vi "DB_LeeEstadoEquipos.vi"(8 "error in (no error)":errorcluster, 11 "db in":T1) -> (0 "error out":errorcluster, 2 "ESTADO_EQUIPOS":string[](array[string]), 3 "db out":T1)   [LabVIEW 2018]
uses:
  <vilib>/addons/database/Connection.llb/Conn ObjectReference.ctl
  <vilib>/Utility/sysdir.llb/System Directory Type.ctl
  <vilib>/Utility/file.llb/Read Delimited Spreadsheet (string).vi
  <vilib>/addons/database/Connection.llb/Conn Execute.vi
  <vilib>/addons/database/Recordset.llb/Rec Fetch Recordset Data (R).vi
  <vilib>/addons/database/Recordset.llb/Rec Destroy - Connection.vi
  <vilib>/addons/database/_DB Variant To Data/Database Variant To Data.xnode
  <vilib>/addons/database/NI_Database_API.lvlib
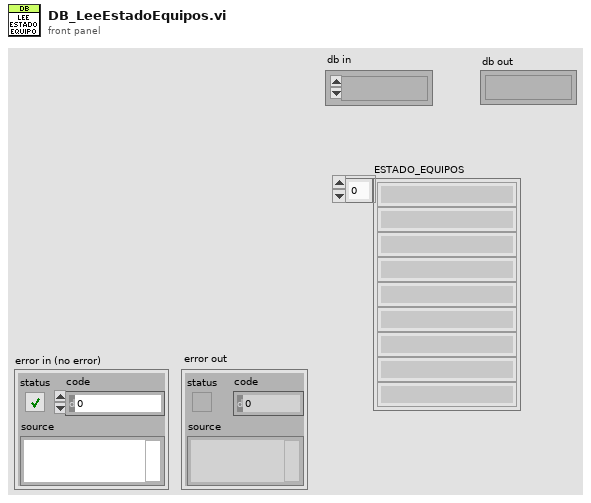
[diagram p1: front panel]
types:
  T1 = typedef "NI_Database_API.lvlib/Conn ObjectReference.ctl" = refnum<k1>
  T2 = typedef "System Directory Type.ctl" = i32
  T3 = typedef "NI_Database_API.lvlib/Rec ObjectReference.ctl" = refnum<k1>
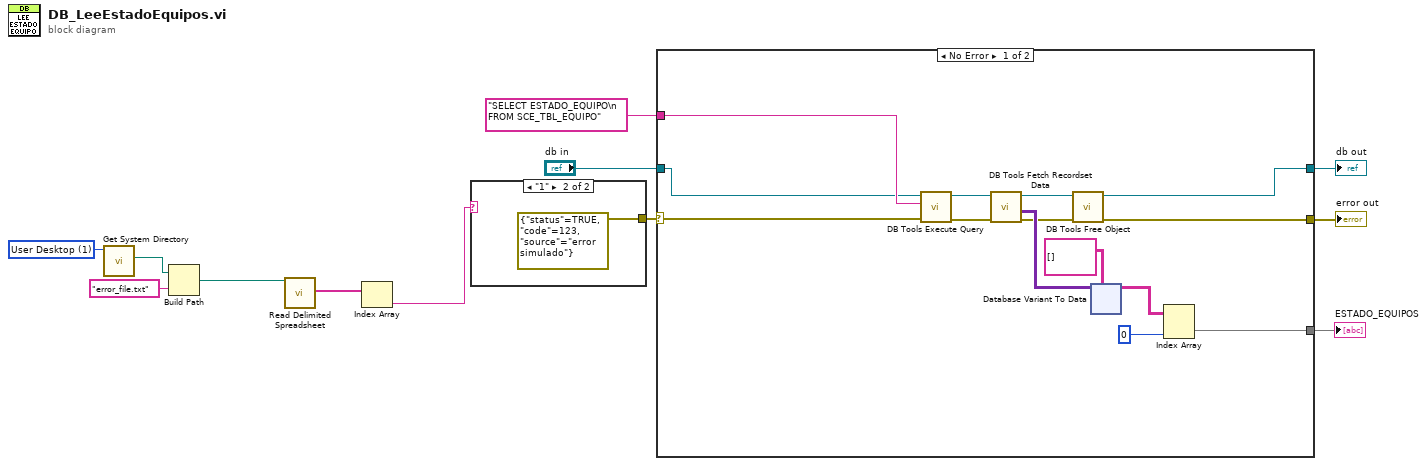
[diagram p0: block diagram]
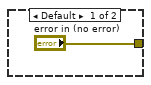
[diagram p2: hidden frame]
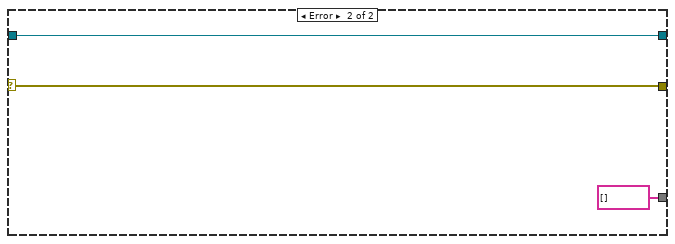
[diagram p3: hidden frame]
diagram:
  w7 = T2 1 items=["User Home"=0, "User Desktop"=1, "User Documents"=2, "User Application Data"=3, "User Preferences"=4, "User Temporary"=5, "Public Documents"=6, "Public Application Data"=7, "Public Preferences"=8, "Public Cache"=13, "System Core Libraries"=9, "System Installed Libraries"=10, "Application Files"=11, "Boot Volume Root"=12] ("system directory type")
  n1 = call <vilib>:"Get System Directory.vi"("system directory type"=w7) -> ("system directory"=w6:path)  [unwired: 10 in]
  n2 = Build Path(base path=w6, name or relative path="error_file.txt") -> (appended path=w4:path)
  n3 = call-poly <vilib>:"Read Delimited Spreadsheet.vi"("file path (dialog if empty)"=w4) -> ("first row"=w3:string[])  [unwired: 9 in, 5 out]
  n4 = Index Array(array=w3) -> (element=w2:string)  [unwired: 1 in]
  n5 = case shown="\"1\"" w2 {
    tunnel: ["error in (no error)" errorcluster {"status"=TRUE, "code"=123, "source"="error simulado"} ("error in (error)")] -> w11
    frame Default {
    }
    frame "1" {
    }
  }
  n6 = case shown="No Error" w11 {
    selector: w11 -> [w26 w75]
    tunnel: [w28 w75] -> w12
    tunnel: "SELECT ESTADO_EQUIPO\n  FROM SCE_TBL_EQUIPO" ("SQL") -> [w25 _]
    tunnel: "db in" -> [w15 w74]
    tunnel: [w17 w74] -> w8
    tunnel: [w16 string[] [] ("data")] -> w1
    frame No Error {
      n7 = call-poly <vilib>:"DB Tools Execute Query.vi"("error in (no error)"=w26, "SQL query"=w25, "connection reference"=w15) -> ("error out"=w27:errorcluster, "recordset reference"=w24:T3)  [unwired: 5 in]
      n8 = call-poly <vilib>:"DB Tools Fetch Recordset Data.vi"("error in (no error)"=w27, "recordset reference"=w24) -> ("error out"=w20:errorcluster, "recordset data"=w21:variant[][], "recordset reference out"=w23:T3)  [unwired: 3 in]
      n9 = call-poly <vilib>:"DB Tools Free Object.vi"("error in (no error)"=w20, "recordset reference"=w23) -> ("error out"=w28:errorcluster, "connection reference"=w17:T1)  [unwired: 8 in]
      n10 = xnode "Database Variant To Data"("database variant"=w21, "type"=string[][] []) -> ("data"=w18:string[][])  [unwired: 1 in, 1 out]
      n11 = Index Array(array=w18, index (col)=0 ("disabled index (col)")) -> (element=w16:string[])  [unwired: 1 in]
    }
    frame Error {
    }
  }
  "error out" <- w12
  "db out" <- w8
  "ESTADO_EQUIPOS" <- w1
